vi "Copy File with Progress Example.vi"() -> ()   [LabVIEW 2016]
uses:
  Copy File DLL/x64/Debug/Copy File DLL.dll
panel:
  in  "Cancel":bool
  out "Update Value (%)":u8
  out "Copy Success?":i32
  in  "Destination":path=path "D:/Microscope-Control/Tools/Copy File with Progress/Test Image File COPY01.dcimg"
  in  "File to Copy":path=path "D:/Microscope-Control/Tools/Copy File with Progress/Test Image File.dcimg"
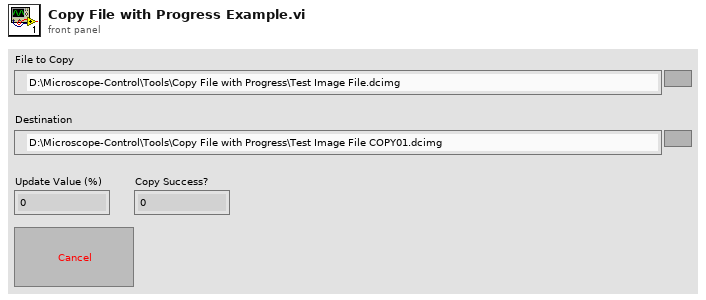
[diagram p1: front panel]
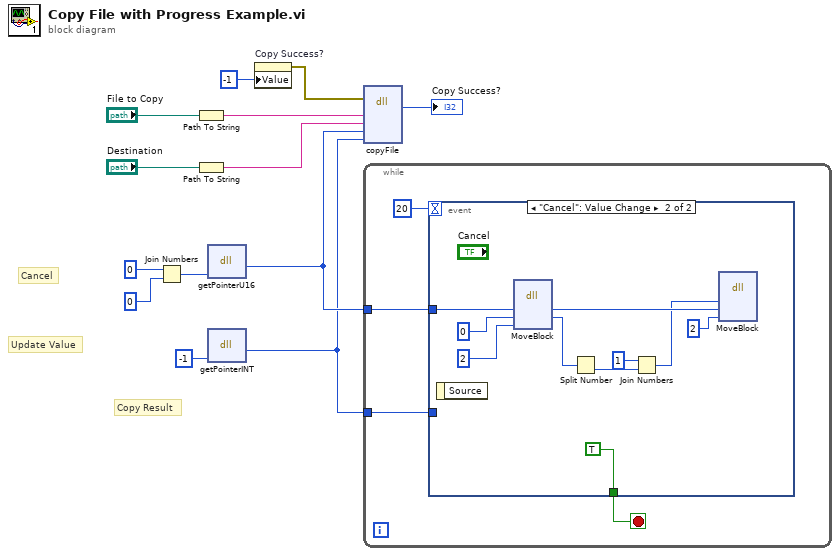
[diagram p0: block diagram]
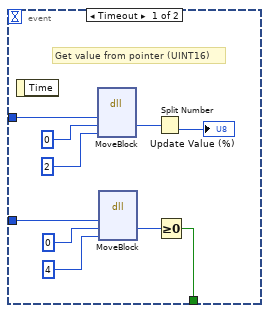
[diagram p2: hidden frame]
diagram:
  # "Copy Result"
  # "Update Value"
  # "Cancel"
  n1 = Join Numbers(hi=u8 0, lo=u8 0) -> ((hi.lo)=w5:u16)
  n2 = Path To String(path="File to Copy") -> (string=w8:string)
  n3 = Path To String(path="Destination") -> (string=w9:string)
  n4 = dll-call lib="D:/Microscope-Control/Tools/Copy File with Progress/Copy File DLL/x64/Debug/Copy File DLL.dll" fn="getPointerU16"("Variable"=w5) -> ("Pointer Value"=w6:u64)  [unwired: 4 in, 2 out]
  n5 = dll-call lib="D:/Microscope-Control/Tools/Copy File with Progress/Copy File DLL/x64/Debug/Copy File DLL.dll" fn="getPointerINT"("Variable"=-1) -> ("Pointer Value"=w1:u64)  [unwired: 4 in, 2 out]
  n6 = property on="Copy Success?" class="DigNum (strict)"("Value"=-1 ("Copy Success?")) -> (error out=w3:errorcluster)  [unwired: 2 in, 1 out]
  n7 = dll-call lib="D:/Microscope-Control/Tools/Copy File with Progress/Copy File DLL/x64/Debug/Copy File DLL.dll" fn="copyFile"(error in=w3, "Source File"=w8, "Destination File"=w9, "Update Value Pointer"=w6, "Copy Result Pointer"=w1) -> ("Success"=→"Copy Success?":i32)  [unwired: 6 in, 2 out]
  n8 = while {
    tunnel: w6 -> [w16]
    tunnel: w1 -> [w15]
    stop <- w14 stop-if-true
    n9 = event shown="[1] \"Cancel\": Value Change" {
      selector: _ -> [_ _]
      dyn-events: _ -> [_ _]
      timeout: 20 -> [_ _]
      tunnel: w16 -> [w24 w33]
      tunnel: w15 -> [w20 _]
      tunnel: [w18 TRUE] -> w14
      event Timeout {
        # "Get value from pointer (UINT16)"
        n10 = event-data() -> ()  [unwired: 1 in, 1 out]
        n11 = dll-call lib="LabVIEW" fn="MoveBlock"("Pointer to Source"=w24, "Destination"=u16 0, "Bytes to Move"=2) -> ("Destination"=w25:u16)  [unwired: 6 in, 2 out]
        n12 = dll-call lib="LabVIEW" fn="MoveBlock"("Pointer to Source"=w20, "Destination"=0, "Bytes to Move"=4) -> ("Destination"=w19:i32)  [unwired: 6 in, 2 out]
        n13 = Split Number(x=w25) -> (lo(x)=→"Update Value (%)":u8)  [unwired: 1 out]
        n14 = Greater Or Equal To 0?(x=w19) -> (x >= 0?=w18:bool)
      }
      event "Cancel": Value Change {
        n15 = event-data() -> ()  [unwired: 1 in, 1 out]
        n16 = dll-call lib="LabVIEW" fn="MoveBlock"("Pointer to Source"=w33, "Destination"=u16 0, "Bytes to Move"=2) -> ("Pointer to Source"=w29:u64, "Destination"=w34:u16)  [unwired: 5 in, 2 out]
        n17 = Split Number(x=w34) -> (lo(x)=w32:u8)  [unwired: 1 out]
        n18 = Join Numbers(hi=u8 1, lo=w32) -> ((hi.lo)=w28:u16)
        n19 = dll-call lib="LabVIEW" fn="MoveBlock"("Source"=w28, "Destination Pointer"=w29, "Bytes to Move"=2) -> ()  [unwired: 7 in, 2 out]
      }
    }
  }
